vi "Stereo - Grid Feature Extraction.vi"(6 "Grid Size":cluster{"X":sgl, "Y":sgl}={"X"=1.0, "Y"=1.0}, 8 "error in (no error)":errorcluster, 9 "Grid Descriptor":cluster{"X":sgl, "Y":sgl, "Unit":T2}={"X"=1.0, "Y"=1.0, "Unit"=enum."Centimeter"}, 10 "Display Image in":T3, 11 "Image in":T3) -> (0 "error out":errorcluster, 1 "Reference Points":T1, 2 "Display Image out":T3, 3 "Image (dup)":T3, 4 "Valid Grid":bool, 5 "Color Palette":cluster{"Red":u8, "Green":u8, "Blue":u8}[](array[cluster]))   [LabVIEW 2014]
doc: "Extracts the features from the input grid image, and creates a display image to display the results with a color palette."
uses:
  <vilib>/vision/Image Controls.llb/IMAQ Image.ctl
  <vilib>/vision/Calibration.llb/Calibration Reference Points.ctl
  Stereo - Calibration Manager Function.ctl
  <vilib>/vision/NI_Vision_Development_Module.lvlib
panel:
  # "Overview: Extracts the features from the input grid image, and creates a display image to display the results with a color palette."
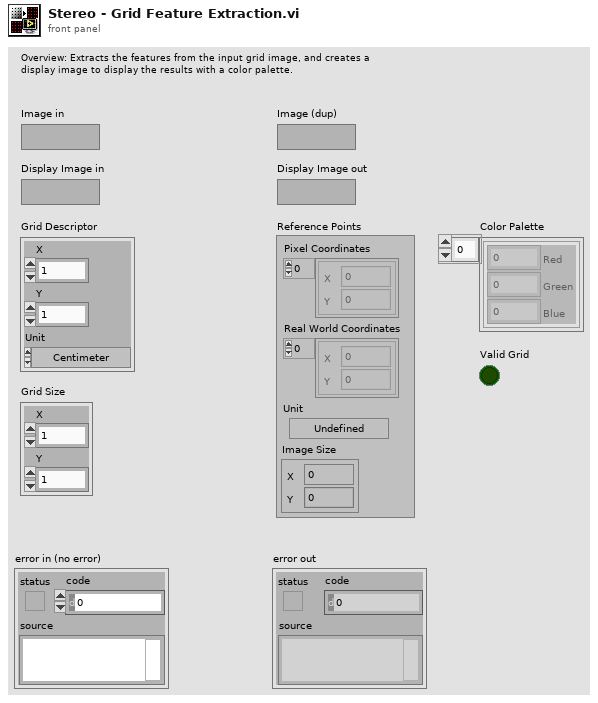
[diagram p1: front panel]
types:
  T1 = typedef "Calibration Reference Points.ctl" = cluster{"Pixel Coordinates":cluster{"X":dbl, "Y":dbl}[], "Real World Coordinates":cluster{"X":dbl, "Y":dbl}[], "Unit":T2, "Image Size":cluster{"X":u32, "Y":u32}}
  T2 = typedef "Image Unit" = enum32{"Undefined", "Angström", "Micrometer", "Millimeter", "Centimeter", "Meter", "Kilometer", "Microinch", "Inch", "Feet", "Nautical miles", "Standard miles", "Steps"}
  T3 = typedef "IMAQ Image.ctl" = refnum<image>
  T4 = typedef "Particle Parameters" = i32
  T5 = cluster{"Measurement Parameter":T4, "Range Lower Value":dbl, "Range Upper Value":dbl, "Range":bool, "Measurement Type":bool}[]
  T6 = enum32{"Average", "Min", "Max", "Clear  if < ", "Clear  if < or =", "Clear  if =", "Clear  if > or =", "Clear  if >"}
  T7 = typedef "Stereo - Calibration Manager Function.ctl" = enum16{"Init", "Add Grid Images", "Get Images", "Dispose"}
  T8 = typedef "Image Type" = u32
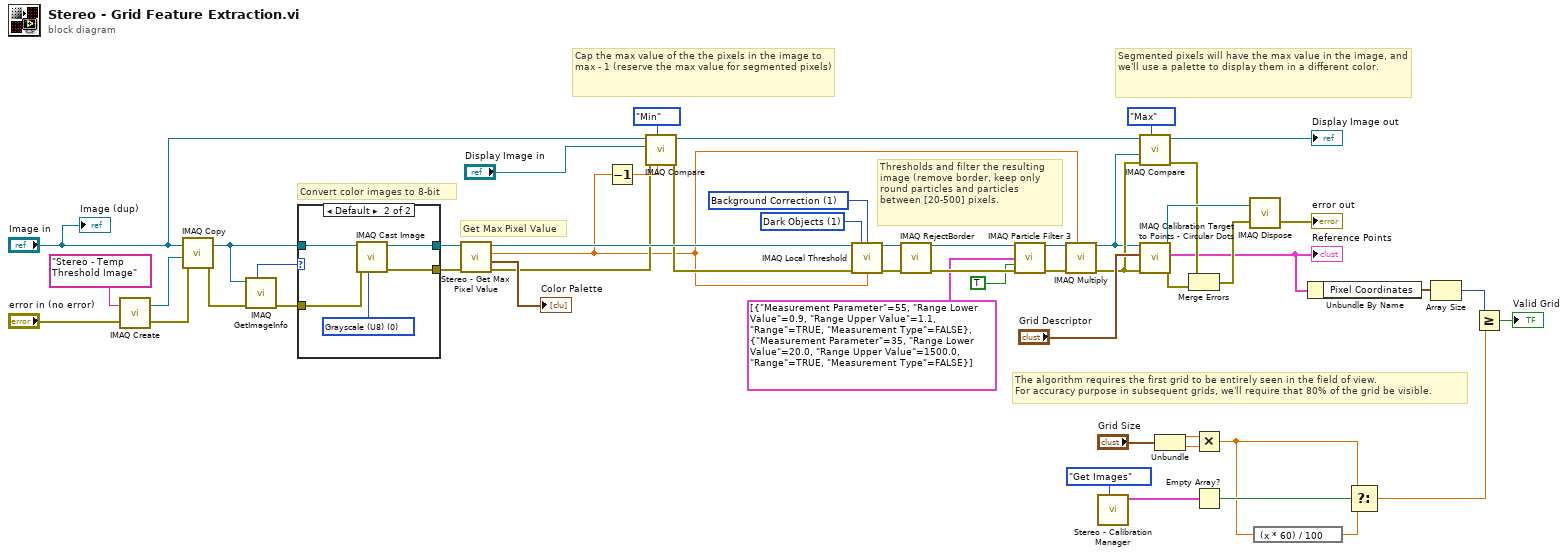
[diagram p0: block diagram]
diagram:
  w33 = u32 1 items=["Niblack", "Background Correction"] ("Method (Niblack)")
  w34 = u32 1 items=["Bright Objects", "Dark Objects"] ("Look For (Bright Objects)")
  # "Convert color images to 8-bit"
  # "Segmented pixels will have the max value in the image, and we'll use a palette to display them in a different color."
  # "Cap the max value of the the pixels in the image to max - 1 (reserve the max value for segmented pixels)"
  # "Thresholds and filter the resulting image (remove border, keep only round particles and particles between [20-500] pixels."
  # "Get Max Pixel Value"
  # "The algorithm requires the first grid to be entirely seen in the field of view.\nFor accuracy purpose in subsequent grids, we'll require that 80% of the grid be visible."
  n1 = call "IMAQ Create"("Image Name"="Stereo - Temp Threshold Image", "error in (no error)"="error in (no error)") -> ("New Image"=w19:T3, "error out"=w18:errorcluster)  [unwired: 2 in, 1 out]
  n2 = call "IMAQ Copy"("error in (no error)"=w18, "Image Dst"=w19, "Image Src"="Image in") -> ("error out"=w17:errorcluster, "Image Dst Out"=w29:T3)  [unwired: 3 out]
  n3 = call "IMAQ GetImageInfo"("error in (no error)"=w17, "Image"=w29) -> ("error out"=w16:errorcluster, "Image Type"=w31:T8)  [unwired: 8 out]
  n4 = case shown="Default" w31 {
    tunnel: w29 -> [w55 w60]
    tunnel: [w55 w59] -> w30
    tunnel: w16 -> [w54 w57]
    tunnel: [w54 w56] -> w11
    frame 0, 1, 7 {
    }
    frame Default {
      w58 = T8 0 items=["Grayscale (U8)", "Grayscale (I16)", "Grayscale (SGL)", "Complex (CSG)", "RGB (U32)", "HSL (U32)", "RGB (U64)", "Grayscale (U16)"] ("Image Type")
      n5 = call "IMAQ Cast Image"("Image Type"=w58, "error in (no error)"=w57, "Image Src"=w60) -> ("error out"=w56:errorcluster, "Image Dst Out"=w59:T3)  [unwired: 3 in, 4 out]
    }
  }
  n6 = call "Stereo - Get Max Pixel Value.vi"("error in (no error)"=w11, "Image"=w30) -> ("error out"=w10:errorcluster, "Color Palette"=→"Color Palette":cluster{"Red":u8, "Green":u8, "Blue":u8}[], "Max Value"=w2:dbl, "Image dup"=w12:T3)  [unwired: 6 out]
  n7 = Decrement(x=w2) -> (x-1=w27:dbl)
  n8 = call "IMAQ Compare"("Constant"=w27, "Operator"=T6."Min", "error in (no error)"=w10, "Image Dst"="Display Image in", "Image Src A"="Image in") -> ("error out"=w9:errorcluster, "Image Dst Out"=w26:T3)  [unwired: 1 in, 4 out]
  n9 = call "IMAQ Local Threshold"("Image Src"=w12, "Look For (Bright Objects)"=w34, "Method (Niblack)"=w33, "error in (no error)"=w9, "Replace Value (1)"=w2) -> ("Image Dst Out"=w24:T3, "error out"=w25:errorcluster)  [unwired: 3 in, 6 out]
  n10 = call "IMAQ RejectBorder"("error in (no error)"=w25, "Image Src"=w24) -> ("error out"=w22:errorcluster, "Image Dst Out"=w23:T3)  [unwired: 2 in, 2 out]
  n11 = call "IMAQ Particle Filter 3"("Image Src"=w23, "Selection Values"=T5 [{"Measurement Parameter"=55, "Range Lower Value"=0.9, "Range Upper Value"=1.1, "Range"=TRUE, "Measurement Type"=FALSE}, {"Measurement Parameter"=35, "Range Lower Value"=20.0, "Range Upper Value"=1500.0, "Range"=TRUE, "Measurement Type"=FALSE}], "Keep/Remove Particles (F)"=TRUE, "error in (no error)"=w22) -> ("Image Dst Out"=w4:T3, "error out"=w6:errorcluster)  [unwired: 5 in, 5 out]
  n12 = call "IMAQ Multiply"("Image Src A"=w4, "Constant"=w2, "error in (no error)"=w6) -> ("Image Dst Out"=w3:T3, "error out"=w5:errorcluster)  [unwired: 2 in, 2 out]
  n13 = call "Stereo - Calibration Manager.vi"("Function"=Stereo_-_Calibration_Manager_Function."Get Images") -> ("Grid Images out"=w36:cluster{"Left Image":T3, "Right Image":T3}[])  [unwired: 2 in, 8 out]
  n14 = call "IMAQ Compare"("Operator"=T6."Max", "error in (no error)"=w5, "Image Src B"=w3, "Image Src A"=w26) -> ("error out"=w7:errorcluster, "Image Dst Out"=→"Display Image out":T3)  [unwired: 2 in, 4 out]
  n15 = call "IMAQ Calibration Target to Points - Circular Dots"("error in (no error)"=w5, "Grid Descriptor"="Grid Descriptor", "Target Image"=w3) -> ("error out"=w15:errorcluster, "Reference Points"=w1:T1, "Target Image (dup)"=w14:T3)  [unwired: 2 in, 4 out]
  "Reference Points" <- w1
  n16 = Unbundle("Grid Size") -> ("X"=w45:sgl, "Y"=w43:sgl)
  n17 = Merge Errors(w7, w15) -> (w8:errorcluster)
  n18 = Multiply(x=w45, y=w43) -> (x*y=w41:sgl)
  n19 = Empty Array?(array=w36) -> (empty?=w42:bool)
  n20 = call "IMAQ Dispose"("Image"=w14, "error in (no error)"=w8) -> ("error out"=→"error out":errorcluster)  [unwired: 1 in, 3 out]
  n21 = expression code="(x * 60) / 100"(w41) -> (w40:sgl)
  n22 = Unbundle By Name(w1) -> ("Pixel Coordinates"=w49:cluster{"X":dbl, "Y":dbl}[])
  n23 = Select(t=w41, s=w42, f=w40) -> (s? t:f=w38:sgl)
  n24 = Array Size(array=w49) -> (size(s)=w39:i32)
  n25 = Greater Or Equal?(x=w39, y=w38) -> (x >= y?=→"Valid Grid":bool)
  "Image (dup)" <- "Image in"
